vi "Resample VR Data.vi"(7 "Memory Size":i32=32768, 11 "Data In":dbl[](array[numeric])) -> (3 "Resampled Data":dbl[](array[numeric]))   [LabVIEW 2011, in "Engine Sim System Explorer.lvlib"]
uses:
  Engine Sim System Explorer.lvlib
  <vilib>/measure/maresamp.llb/Resample Waveform (continuous).vi
  <vilib>/measure/NI_MAPro.lvlib
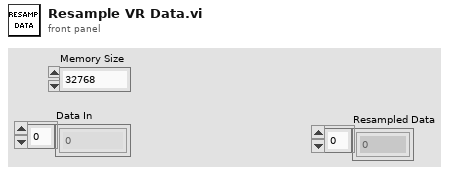
[diagram p1: front panel]
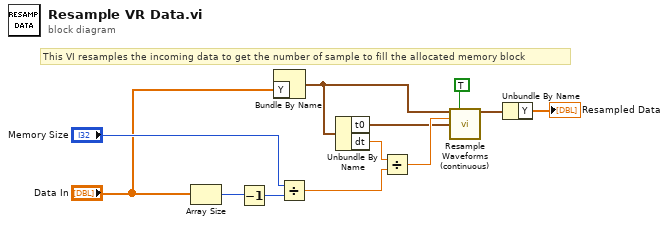
[diagram p0: block diagram]
diagram:
  # "This VI resamples the incoming data to get the number of sample to fill the allocated memory block"
  n1 = Array Size(array="Data In") -> (size(s)=w11:i32)
  n2 = Decrement(x=w11) -> (x-1=w12:i32)
  n3 = Bundle By Name("Y"="Data In") -> (w9:waveform(dbl))  [unwired: 1 in]
  n4 = Divide(x="Memory Size", y=w12) -> (x/y=w7:dbl)
  n5 = Unbundle By Name(w9) -> ("t0"=w5:timestamp, "dt"=w6:dbl)
  n6 = Divide(x=w6, y=w7) -> (x/y=w8:dbl)
  n7 = call-poly <vilib>:"Resample Waveforms (continuous).vi"("waveform in"=w9, "reset"=TRUE, "dt"=w8, "t0"=w5) -> ("resampled waveform out"=w3:waveform(dbl))  [unwired: 7 in, 4 out]
  n8 = Unbundle By Name(w3) -> ("Y"=→"Resampled Data":dbl[])
